vi "BMI160_AccGyr.vi"(1 "Offset":sgl, 2 "Range":sgl=1.0, 3 "Word (string, big endian)":string="\u0000\u0000") -> (0 "eng val":sgl=23.0)   [LabVIEW 2015]
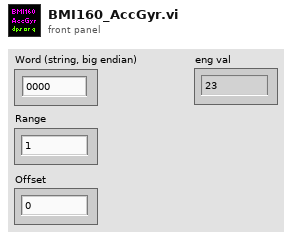
[diagram p1: front panel]
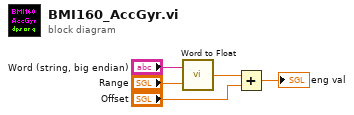
[diagram p0: block diagram]
diagram:
  n1 = call "Word to Float.vi"("Range"="Range", "Word (string, big endian)"="Word (string, big endian)") -> ("float32 out"=w4:sgl)
  n2 = Add(x=w4, y="Offset") -> (x+y=→"eng val":sgl)
